vi "Open.vi"(8 "error in (no error)":errorcluster, 10 "address":string, 11 "Instrument.TC in":refnum<class "Instrument.TC.lvclass">) -> (0 "error out":errorcluster, 3 "Instrument.TC out":refnum<class "Instrument.TC.lvclass">)   [LabVIEW 2019, in "Instrument.TC.lvclass"]
uses:
  Instrument.TC.lvclass
  <userlib>/LevyLab/Instrument Framework/Instrument Types/Cryostat/Instrument.Cryostat.lvclass
  <userlib>/LevyLab/Instrument Framework/SMOs/Instrument/Instrument.lvclass
  C:/Program Files (x86)/National Instruments/LabVIEW 2019/user.lib/LevyLab/Instrument Framework/Instrument Types/Cryostat/Instrument.Cryostat.lvclass
  C:/Program Files (x86)/National Instruments/LabVIEW 2019/user.lib/LevyLab/Instrument Framework/SMOs/Instrument/Instrument.lvclass
  C:/Program Files (x86)/National Instruments/LabVIEW 2019/vi.lib/JKI/JKI SMO/SMO/SMO.lvclass
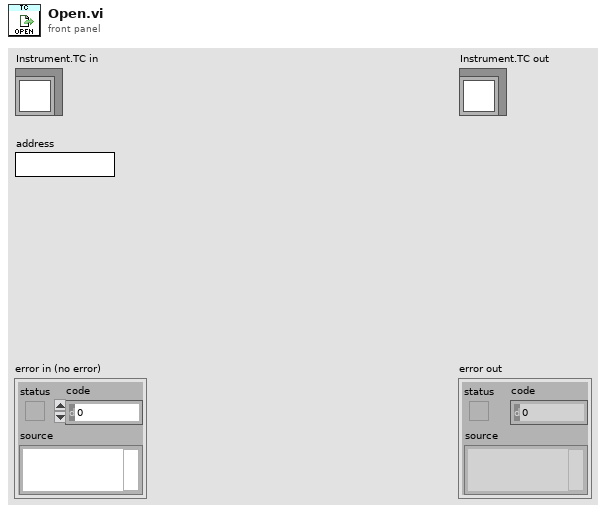
[diagram p1: front panel]
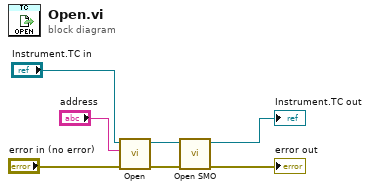
[diagram p0: block diagram]
diagram:
  n1 = call-parent "Open.vi"("error in (no error)"="error in (no error)", "address"="address", "Instrument in"="Instrument.TC in") -> ("error out"=w1:errorcluster, "Instrument out"=w4:refnum<class "Instrument.TC.lvclass">)  [unwired: 7 in]
  n2 = call <userlib>:"Open SMO.vi"("error in (no error)"=w1, "Instrument in"=w4) -> ("error out"=→"error out":errorcluster, "Instrument out"=→"Instrument.TC out":refnum<class "Instrument.TC.lvclass">)  [unwired: 8 in]
